vi "_Truncate Path.vi"(4 "Length (70)":i32=70, 7 "Path":path) -> (3 "String":string)   [LabVIEW 2012]
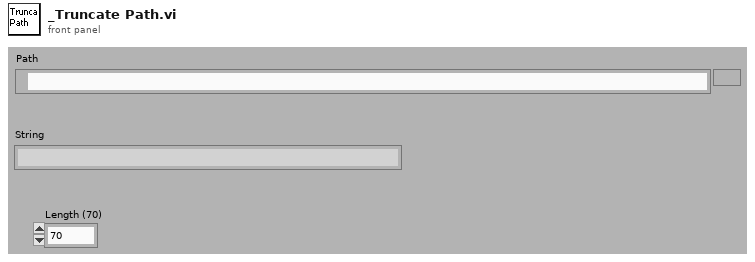
[diagram p1: front panel]
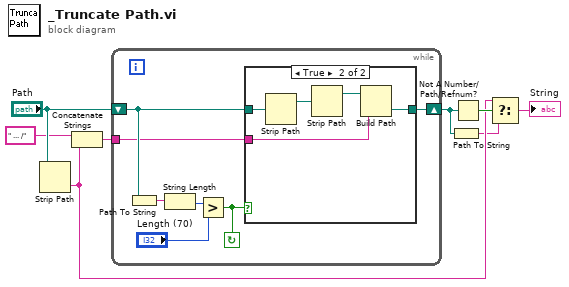
[diagram p0: block diagram]
diagram:
  n1 = Strip Path(path="Path") -> (name=w3:string)  [unwired: 1 out]
  n2 = Concatenate Strings(" ... /" ("Substring"), w3) -> (w6:string)
  n3 = while {
    tunnel: w6 -> [w9]
    shift-left: "Path" -> [w11]
    shift-right: [w10] -> w5
    stop <- w12 continue-if-true
    n4 = Path To String(path=w11) -> (string=w15:string)
    n5 = String Length(string=w15) -> (length=w14:i32)
    n6 = Greater?(x=w14, y="Length (70)") -> (0:w12:bool)
    n7 = case shown="True" w12 {
      tunnel: w11 -> [w16 w21]
      tunnel: [w16 w17] -> w10
      tunnel: w9 -> [_ w18]
      frame False {
      }
      frame True {
        n8 = Strip Path(path=w21) -> (stripped path=w20:path)  [unwired: 1 out]
        n9 = Strip Path(path=w20) -> (stripped path=w19:path)  [unwired: 1 out]
        n10 = Build Path(base path=w19, name or relative path=w18) -> (appended path=w17:path)
      }
    }
  }
  n11 = Path To String(path=w5) -> (string=w2:string)
  n12 = Not A Number/Path/Refnum?(number/path/refnum=w5) -> (NaN/Path/Refnum?=w4:bool)
  n13 = Select(t=w3, s=w4, f=w2) -> (s? t:f=→"String":string)
